vi "DeleteDup.vi"(11 "Array in":i32[](array[numeric])) -> (3 "Array out":i32[](array[numeric]))   [LabVIEW 2017]
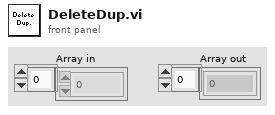
[diagram p1: front panel]
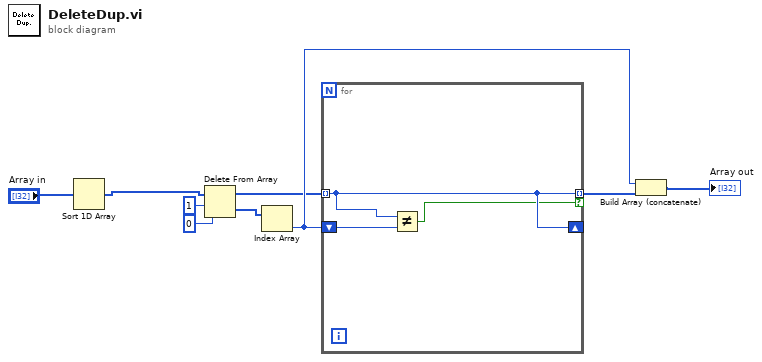
[diagram p0: block diagram]
diagram:
  n1 = Sort 1D Array(array="Array in") -> (sorted array=w9:i32[])
  n2 = Delete From Array(array=w9, length=1, index=0) -> (deleted portion=w3:i32[], array with subset deleted=w4:i32[])
  n3 = Index Array(array=w3) -> (element=w6:i32)  [unwired: 1 in]
  n4 = for {
    shift-right: [w11] -> _
    shift-left: w6 -> [w12]
    tunnel: w4 -> [w11] mode=indexing
    tunnel: [w11] -> w5 mode=indexing if=w10
    n5 = Not Equal?(x=w11, y=w12) -> (x != y?=w10:bool)
  }
  n6 = Build Array (concatenate)(w6, w5) -> (→"Array out":i32[])
